vi "Panel Stop Condition.vi"() -> (3 "Enable Time Limit Out":bool, 4 "Time Limit(s) Out":dbl=5400.0 format="%<%H:%M:%S>t", 6 "Enable RMC Limit Out":bool, 8 "RMC Limit Out":dbl=2.0, 10 "Enable Stop On Power Off Out":bool=TRUE, 14 "Power Off Time(samples) Out":i32=60, 15 "Power Off Check":bool[](array[boolean]))   [LabVIEW 2012]
panel:
  in  "stop":bool
  in  "Time Limit(HH:MM:SS)":dbl=5400.0 format="%<%H:%M:%S>t"
  in  "Time Below Set Minimum Wattage":i32=15
  in  "Autoterminate at End of Cycle":bool=TRUE
  in  "RMC Limit":dbl=2.0
  in  "Enable RMC Limit":bool
  in  "Enable Time Limit":bool
  # "Stop Condition"
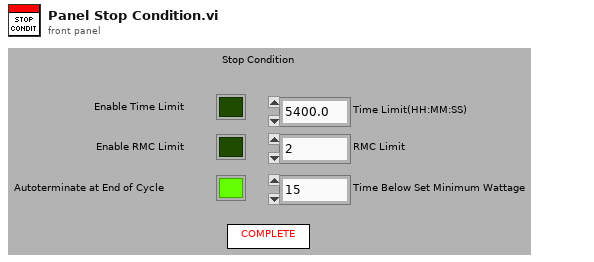
[diagram p1: front panel]
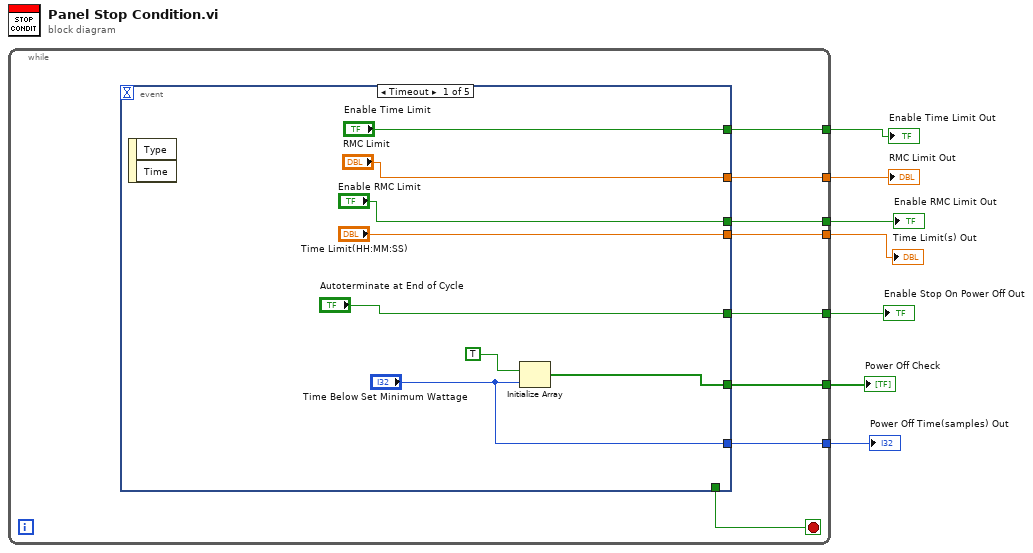
[diagram p0: block diagram]
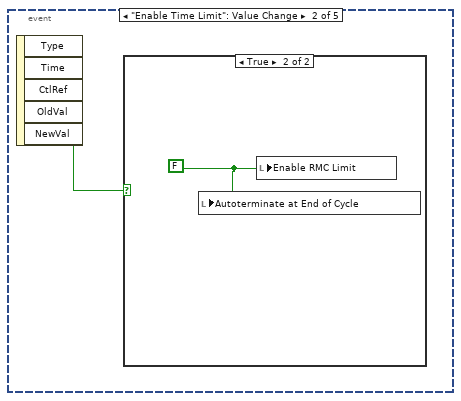
[diagram p2: hidden frame]
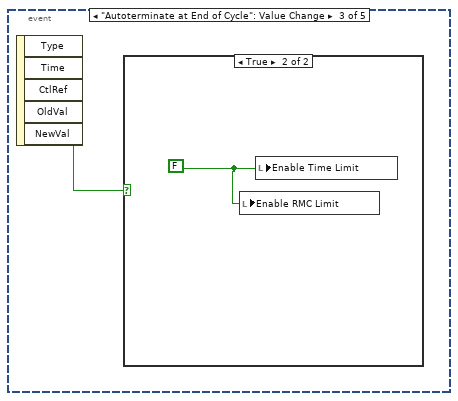
[diagram p4: hidden frame]
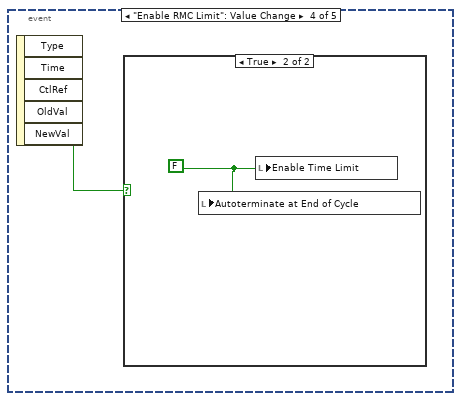
[diagram p6: hidden frame]
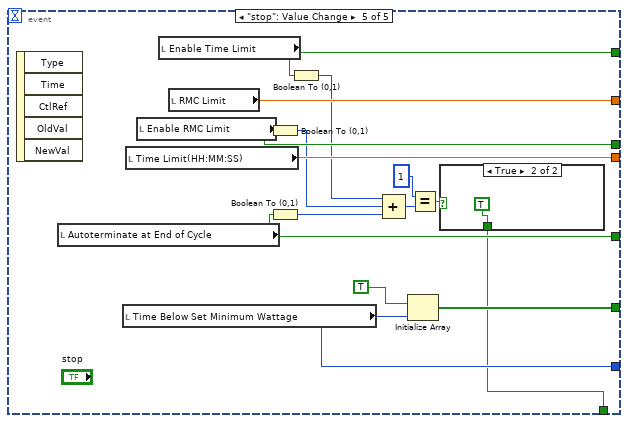
[diagram p8: hidden frame]
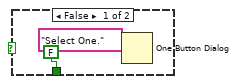
[diagram p9: hidden frame]
diagram:
  n1 = while {
    tunnel: [w15] -> w7
    tunnel: [w14] -> w6
    tunnel: [w13] -> w5
    tunnel: [w12] -> w4
    tunnel: [w11] -> w3
    tunnel: [w10] -> w2
    tunnel: [w9] -> w1
    stop <- w8 stop-if-true
    n2 = event shown="[0] Timeout" {
      selector: _ -> [_ _ _ _ _]
      dyn-events: _ -> [_ _ _ _ _]
      timeout: _ -> [_ _ _ _ _]
      tunnel: [w22 _ _ _ w44] -> w15
      tunnel: ["Enable Time Limit" _ _ _ w39] -> w14
      tunnel: ["RMC Limit" _ _ _ w43] -> w13
      tunnel: ["Enable RMC Limit" _ _ _ w38] -> w12
      tunnel: ["Autoterminate at End of Cycle" _ _ _ w37] -> w11
      tunnel: ["Time Limit(HH:MM:SS)" _ _ _ w42] -> w10
      tunnel: ["Time Below Set Minimum Wattage" _ _ _ w41] -> w9
      tunnel: [_ _ _ _ w31] -> w8
      event Timeout {
        n3 = event-data() -> ()  [unwired: 1 in, 2 out]
        n4 = Initialize Array(TRUE ("Init Complete"), "Time Below Set Minimum Wattage") -> (w22:bool[])
      }
      event "Enable Time Limit": Value Change {
        n5 = event-data() -> ("NewVal"=w24:bool)  [unwired: 1 in, 4 out]
        n6 = case shown="True" w24 {
          frame False {
          }
          frame True {
            w25 = FALSE ("Enable RMC Limit 2")
            n7 = local write "Autoterminate at End of Cycle"(w25) -> ()
            n8 = local write "Enable RMC Limit"(w25) -> ()
          }
        }
      }
      event "Autoterminate at End of Cycle": Value Change {
        n9 = event-data() -> ("NewVal"=w26:bool)  [unwired: 1 in, 4 out]
        n10 = case shown="True" w26 {
          frame False {
          }
          frame True {
            w27 = FALSE ("Enable RMC Limit 2")
            n11 = local write "Enable RMC Limit"(w27) -> ()
            n12 = local write "Enable Time Limit"(w27) -> ()
          }
        }
      }
      event "Enable RMC Limit": Value Change {
        n13 = event-data() -> ("NewVal"=w28:bool)  [unwired: 1 in, 4 out]
        n14 = case shown="True" w28 {
          frame False {
          }
          frame True {
            w29 = FALSE ("Enable RMC Limit 2")
            n15 = local write "Autoterminate at End of Cycle"(w29) -> ()
            n16 = local write "Enable Time Limit"(w29) -> ()
          }
        }
      }
      event "stop": Value Change {
        n17 = event-data() -> ()  [unwired: 1 in, 5 out]
        n18 = local read "Autoterminate at End of Cycle"() -> (w37:bool)
        n19 = local read "Time Below Set Minimum Wattage"() -> (w41:i32)
        n20 = local read "Time Limit(HH:MM:SS)"() -> (w42:dbl)
        n21 = local read "Enable RMC Limit"() -> (w38:bool)
        n22 = local read "Enable Time Limit"() -> (w39:bool)
        n23 = local read "RMC Limit"() -> (w43:dbl)
        n24 = Boolean To (0,1)(Boolean=w38) -> (0, 1=w35:i16)
        n25 = Boolean To (0,1)(Boolean=w37) -> (0, 1=w34:i16)
        n26 = Boolean To (0,1)(Boolean=w39) -> (0, 1=w36:i16)
        n27 = Compound Arithmetic op=ADD(w36, w35, w34) -> (w33:i16)
        n28 = Initialize Array(TRUE ("Init Complete"), w41) -> (w44:bool[])
        n29 = Equal?(x=i16 1, y=w33) -> (x = y?=w30:bool)
        n30 = case shown="True" w30 {
          tunnel: [FALSE ("Init Complete") TRUE ("Init Complete")] -> w31
          frame False {
            n31 = One Button Dialog(message="Select One.") -> ()  [unwired: 1 in, 1 out]
          }
          frame True {
          }
        }
      }
    }
  }
  "Power Off Check" <- w7
  "Enable Time Limit Out" <- w6
  "RMC Limit Out" <- w5
  "Enable RMC Limit Out" <- w4
  "Time Limit(s) Out" <- w2
  "Enable Stop On Power Off Out" <- w3
  "Power Off Time(samples) Out" <- w1
